vi "CRYIntermodulation PairSum Calc.vi"(8 "Is IEC?":bool, 9 "Order Array":dbl[](array[numeric]), 10 "Data Array":dbl[](array[numeric]), 11 "Type":u32) -> (3 "PairSum Array":dbl[](array[numeric]))   [LabVIEW 2013]
panel:
  # "By The Sum of Plus & Minus Pair,\nCalculating the Power Sum."
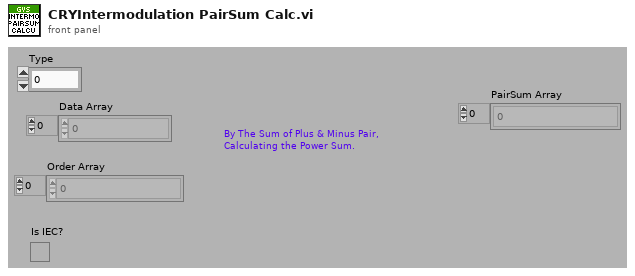
[diagram p1: front panel]
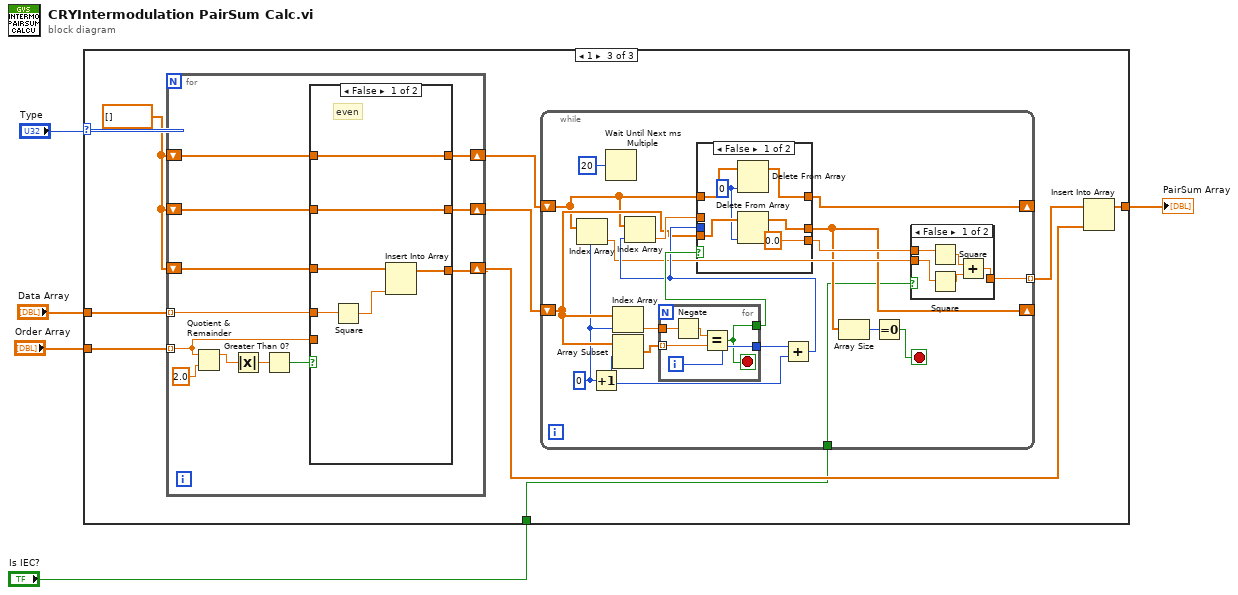
[diagram p0: block diagram]
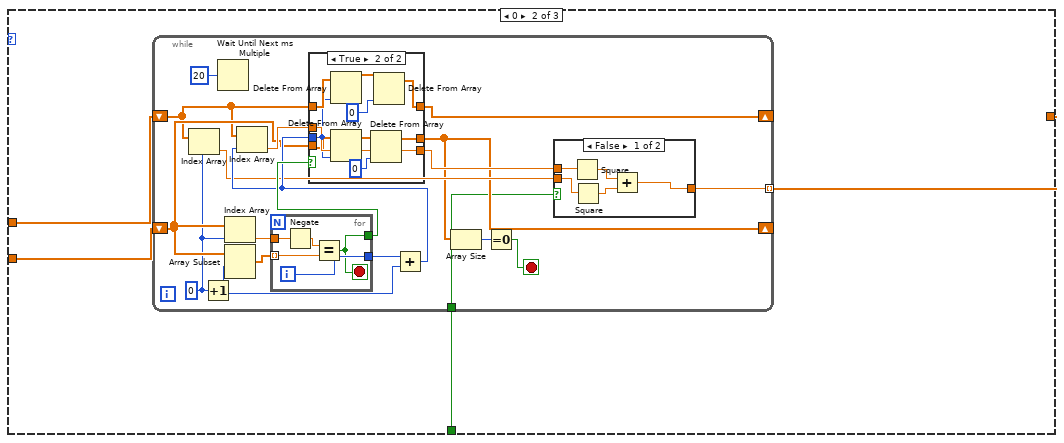
[diagram p3: hidden frame]
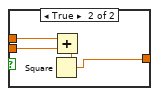
[diagram p4: hidden frame]
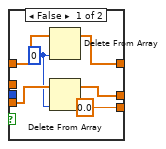
[diagram p5: hidden frame]
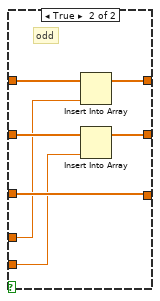
[diagram p6: hidden frame]
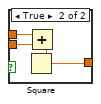
[diagram p7: hidden frame]
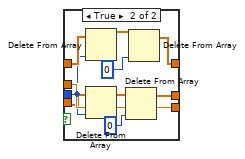
[diagram p8: hidden frame]
diagram:
  n1 = case shown="1" "Type" {
    tunnel: [_ w7 w62] -> w5
    tunnel: "Data Array" -> [_ w9 w67]
    tunnel: "Order Array" -> [_ w8 w66]
    tunnel: "Is IEC?" -> [_ w6 w59]
    frame Default {
    }
    frame 0 {
      n2 = while {
        shift-right: [w23] -> _
        shift-left: w9 -> [w14]
        tunnel: [w19] -> w7 mode=indexing
        shift-right: [w11] -> _
        shift-left: w8 -> [w17]
        tunnel: w6 -> [w10]
        stop <- w12 stop-if-true
        w15 = u32 0 ("millisecond multiple")
        n3 = Index Array(array=w14, index=w15) -> (element=w20:dbl)
        n4 = Increment(x=w15) -> (x+1=w26:u32)
        n5 = Wait Until Next ms Multiple(millisecond multiple=u32 20) -> ()  [unwired: 1 out]
        n6 = Index Array(array=w17, index=w15) -> (element=w16:dbl)
        n7 = Array Subset(array=w17, index=w26) -> (w28:dbl[])  [unwired: 1 in]
        n8 = for {
          tunnel: w28 -> [w56] mode=indexing
          tunnel: w16 -> [w58]
          tunnel: [w55] -> w27
          tunnel: [w54] -> w25
          i -> [w55]
          stop <- w54 stop-if-true
          n9 = Negate(x=w58) -> (-x=w57:dbl)
          n10 = Equal?(x=w57, y=w56) -> (x = y?=w54:bool)
        }
        n11 = Add(x=w27, y=w26) -> (x+y=w22:u32)
        n12 = Index Array(array=w14, index=w22) -> (element=w24:dbl)
        n13 = case shown="True" w25 {
          tunnel: w24 -> [_ w53]
          tunnel: [0.0 ("y") w53] -> w21
          tunnel: [w41 w48] -> w23
          tunnel: w14 -> [w42 w52]
          tunnel: w22 -> [_ w47]
          tunnel: w17 -> [w40 w50]
          tunnel: [w39 w45] -> w11
          frame False {
            w38 = 0 ("index")
            n14 = Delete From Array(array=w42, index=w38) -> (array with subset deleted=w41:dbl[])  [unwired: 1 in, 1 out]
            n15 = Delete From Array(array=w40, index=w38) -> (array with subset deleted=w39:dbl[])  [unwired: 1 in, 1 out]
          }
          frame True {
            n16 = Delete From Array(array=w52, index=w47) -> (array with subset deleted=w51:dbl[])  [unwired: 1 in, 1 out]
            n17 = Delete From Array(array=w50, index=w47) -> (array with subset deleted=w49:dbl[])  [unwired: 1 in, 1 out]
            n18 = Delete From Array(array=w49, index=0) -> (array with subset deleted=w45:dbl[])  [unwired: 1 in, 1 out]
            n19 = Delete From Array(array=w51, index=0) -> (array with subset deleted=w48:dbl[])  [unwired: 1 in, 1 out]
          }
        }
        n20 = Array Size(array=w11) -> (size(s)=w13:i32)
        n21 = Equal To 0?(x=w13) -> (x = 0?=w12:bool)
        n22 = case shown="False" w10 {
          tunnel: w21 -> [w33 w37]
          tunnel: w20 -> [w32 w36]
          tunnel: [w29 w34] -> w19
          frame False {
            n23 = Square(x=w33) -> (x^2=w31:dbl)
            n24 = Square(x=w32) -> (x^2=w30:dbl)
            n25 = Add(x=w31, y=w30) -> (x+y=w29:dbl)
          }
          frame True {
            n26 = Add(x=w37, y=w36) -> (x+y=w35:dbl)
            n27 = Square(x=w35) -> (x^2=w34:dbl)
          }
        }
      }
    }
    frame 1 {
      w65 = dbl[] [] ("subarray")
      n28 = for {
        tunnel: w67 -> [w70] mode=indexing
        tunnel: w66 -> [w68] mode=indexing
        shift-right: [w74] -> w64
        shift-left: w65 -> [w75]
        shift-right: [w72] -> w63
        shift-left: w65 -> [w73]
        shift-right: [w69] -> w61
        shift-left: w65 -> [w71]
        n29 = Quotient & Remainder(x=w68, y=2.0) -> (x-y*floor(x/y)=w77:dbl)  [unwired: 1 out]
        n30 = Absolute Value(x=w77) -> (abs(x)=w79:dbl)
        n31 = Greater Than 0?(x=w79) -> (x > 0?=w76:bool)
        n32 = case shown="False" w76 {
          tunnel: w75 -> [w85 w91]
          tunnel: [w85 w87] -> w74
          tunnel: w73 -> [w84 w90]
          tunnel: [w84 w86] -> w72
          tunnel: w71 -> [w82 w92]
          tunnel: w70 -> [w83 w89]
          tunnel: [w80 w92] -> w69
          tunnel: w68 -> [_ w88]
          frame False {
            # "even"
            n33 = Square(x=w83) -> (x^2=w81:dbl)
            n34 = Insert Into Array(array=w82, new element=w81) -> (w80:dbl[])  [unwired: 1 in]
          }
          frame True {
            # "odd"
            n35 = Insert Into Array(array=w91, new element=w89) -> (w87:dbl[])  [unwired: 1 in]
            n36 = Insert Into Array(array=w90, new element=w88) -> (w86:dbl[])  [unwired: 1 in]
          }
        }
      }
      n37 = while {
        shift-right: [w106] -> _
        shift-left: w64 -> [w97]
        tunnel: [w102] -> w60 mode=indexing
        shift-right: [w94] -> _
        shift-left: w63 -> [w100]
        tunnel: w59 -> [w93]
        stop <- w95 stop-if-true
        w98 = u32 0 ("millisecond multiple")
        n38 = Index Array(array=w97, index=w98) -> (element=w103:dbl)
        n39 = Increment(x=w98) -> (x+1=w109:u32)
        n40 = Wait Until Next ms Multiple(millisecond multiple=u32 20) -> ()  [unwired: 1 out]
        n41 = Index Array(array=w100, index=w98) -> (element=w99:dbl)
        n42 = Array Subset(array=w100, index=w109) -> (w111:dbl[])  [unwired: 1 in]
        n43 = for {
          tunnel: w111 -> [w139] mode=indexing
          tunnel: w99 -> [w141]
          tunnel: [w138] -> w110
          tunnel: [w137] -> w108
          i -> [w138]
          stop <- w137 stop-if-true
          n44 = Negate(x=w141) -> (-x=w140:dbl)
          n45 = Equal?(x=w140, y=w139) -> (x = y?=w137:bool)
        }
        n46 = Add(x=w110, y=w109) -> (x+y=w105:u32)
        n47 = Index Array(array=w97, index=w105) -> (element=w107:dbl)
        n48 = case shown="False" w108 {
          tunnel: w107 -> [_ w136]
          tunnel: [0.0 ("y") w136] -> w104
          tunnel: [w124 w131] -> w106
          tunnel: w97 -> [w125 w135]
          tunnel: w105 -> [_ w130]
          tunnel: w100 -> [w123 w133]
          tunnel: [w122 w128] -> w94
          frame False {
            w121 = 0 ("index")
            n49 = Delete From Array(array=w125, index=w121) -> (array with subset deleted=w124:dbl[])  [unwired: 1 in, 1 out]
            n50 = Delete From Array(array=w123, index=w121) -> (array with subset deleted=w122:dbl[])  [unwired: 1 in, 1 out]
          }
          frame True {
            n51 = Delete From Array(array=w135, index=w130) -> (array with subset deleted=w134:dbl[])  [unwired: 1 in, 1 out]
            n52 = Delete From Array(array=w133, index=w130) -> (array with subset deleted=w132:dbl[])  [unwired: 1 in, 1 out]
            n53 = Delete From Array(array=w132, index=0) -> (array with subset deleted=w128:dbl[])  [unwired: 1 in, 1 out]
            n54 = Delete From Array(array=w134, index=0) -> (array with subset deleted=w131:dbl[])  [unwired: 1 in, 1 out]
          }
        }
        n55 = Array Size(array=w94) -> (size(s)=w96:i32)
        n56 = Equal To 0?(x=w96) -> (x = 0?=w95:bool)
        n57 = case shown="False" w93 {
          tunnel: w104 -> [w116 w120]
          tunnel: w103 -> [w115 w119]
          tunnel: [w112 w117] -> w102
          frame False {
            n58 = Square(x=w116) -> (x^2=w113:dbl)
            n59 = Square(x=w115) -> (x^2=w114:dbl)
            n60 = Add(x=w113, y=w114) -> (x+y=w112:dbl)
          }
          frame True {
            n61 = Add(x=w120, y=w119) -> (x+y=w118:dbl)
            n62 = Square(x=w118) -> (x^2=w117:dbl)
          }
        }
      }
      n63 = Insert Into Array(array=w60, new element=w61) -> (w62:dbl[])  [unwired: 1 in]
    }
  }
  "PairSum Array" <- w5
